vi "dsdll_basic_demo.vi"() -> ()   [LabVIEW 2013, in "dsdll.lvlib"]
doc: "Simple DSDLL demo. Allows to record waveform from selected source and than play it as loop."
uses:
  dsdll.lvlib
  dsdll_instance.ctl
  dsdll_device_record.ctl
  dsdll_format.ctl
  dsdll_sample_format.ctl
  output/dsdll_output_write_auto_float32.vi
  capture/dsdll_capture_wave_auto_float32.vi
panel:
  in  "gui refresh":i32=50 caption="GUI refresh [ms]"
  out "dsdll.dll version string":string
  out "play stat":i32(slide) scale=0.0..100.0
  out "invalid DSDLL instance handle?":bool
  out "output device ok?":bool
  out "output buffer ok?":bool
  out "input capture ok?":bool
  out "rec stat":i32(slide) scale=0.0..100.0
  out "stat str":string caption="Capture progress"
  out "is capturing?":bool
  in  "btn rec abort":bool
  out "record":sgl[][](graph)
  out "rec len out":u32 caption="Recorded samples"
  out "Time stamp [s]":dbl
  in  "btn rec":bool
  in  "btn stop":bool
  out "sound data":sgl[][](array[numeric])
  in  "format":T1={"sample rate [Hz]"=48000, "out channels"=1, "inp channels"=1, "format"=enum."IEEE float 32"} caption="Wave format"
  in  "btn close":bool
  in  "btn open":bool
  in  "btn exit":bool
  in  "rec len":u32=96000 caption="Samples count"
  in  "devs capt":u16(ring) caption="Capture devices" items=["Primarni ovladac pro digitalizaci zvuku", "Mikrofon (Zvukove zarizeni High Definition Audio)"]
  in  "devs out":u16(ring) caption="Output devices" items=["Primarni ovladac zvuku", "Reproduktory (Zvukove zarizeni High Definition Audio)"]
  in  "btn play":bool
  in  "btn enum":bool
  out "error out":errorcluster caption="Error out"
  out "dsdll":T3
  # "DirectSound DLL demo"
  # "1) select in/out devices\n2) select sample format\n3) open DSDLL instace\n4) record waveform\n5) play captured wave"
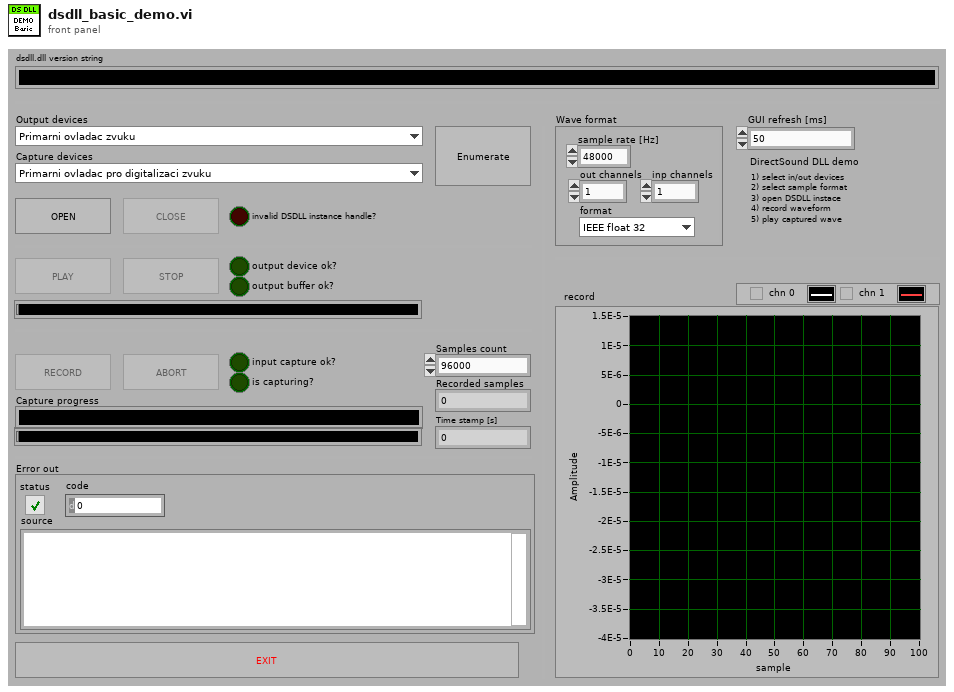
[diagram p1: front panel]
types:
  T1 = typedef "dsdll.lvlib/dsdll_format.ctl" = cluster{"sample rate [Hz]":u32, "out channels":u16, "inp channels":u16, "format":T2}
  T2 = typedef "dsdll.lvlib/dsdll_sample_format.ctl" = enum16{"IEEE float 32", "PCM 16 bit"}
  T3 = typedef "dsdll.lvlib/dsdll_instance.ctl" = cluster{"dsdll path":path, "dsdll handle":u8[], "output devices":T4[], "capture devices":T4[]}
  T4 = typedef "dsdll.lvlib/dsdll_device_record.ctl" = cluster{"guid":u8[], "name":string}
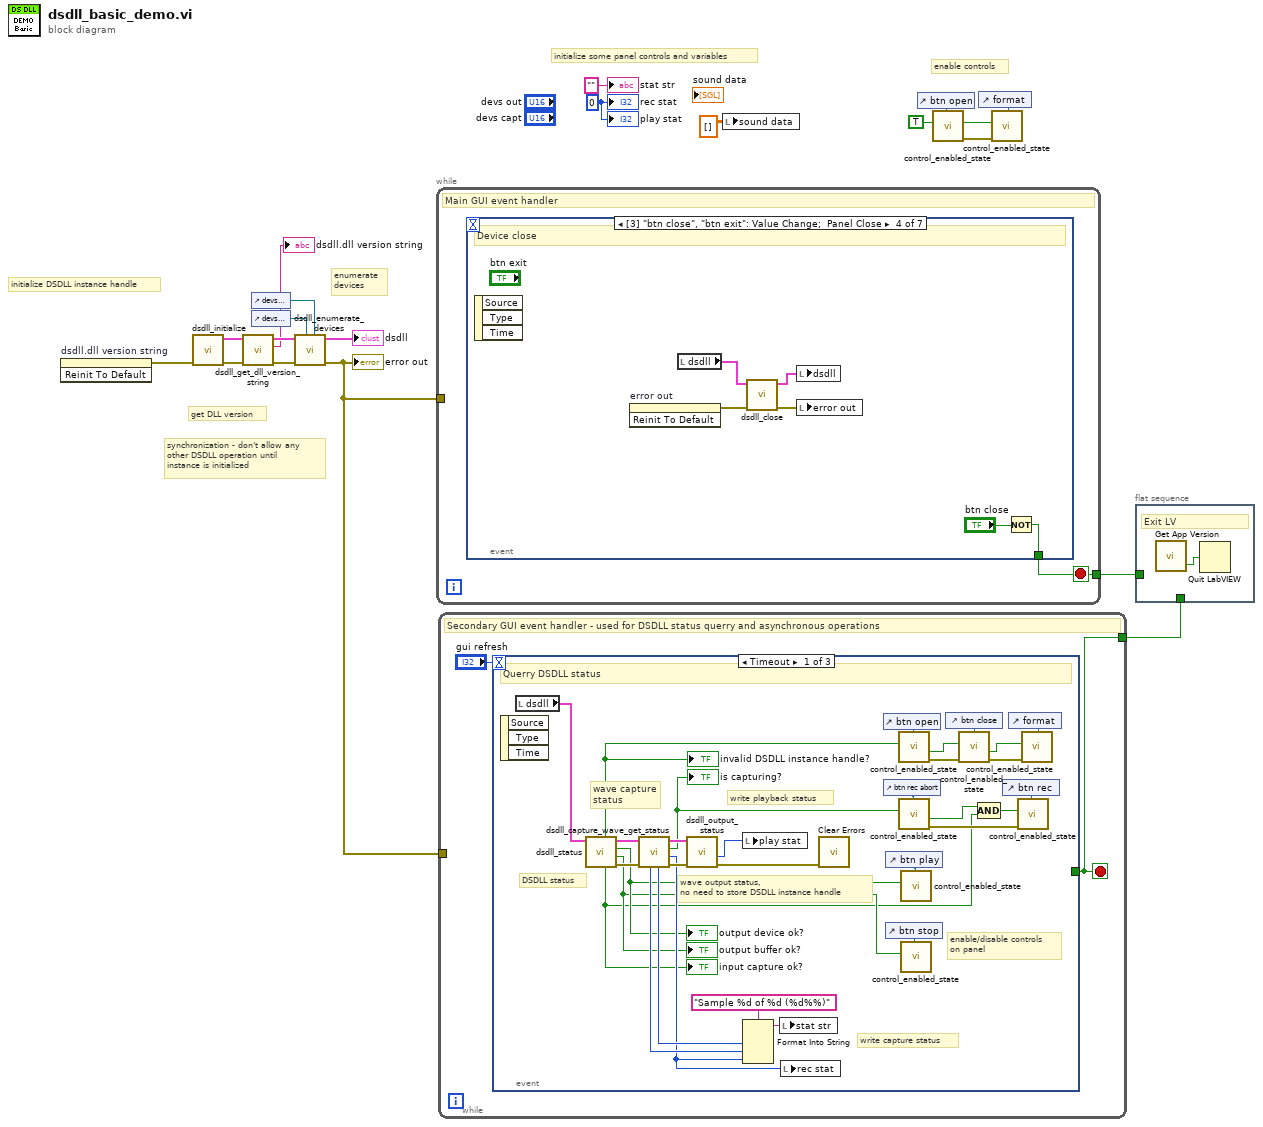
[diagram p0: block diagram]
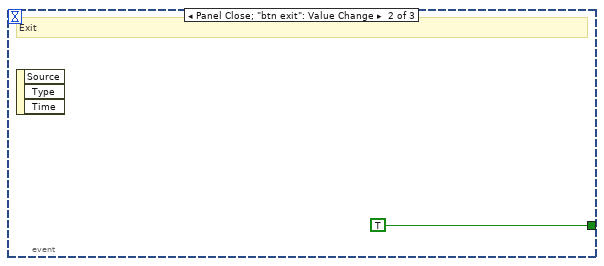
[diagram p2: hidden frame]
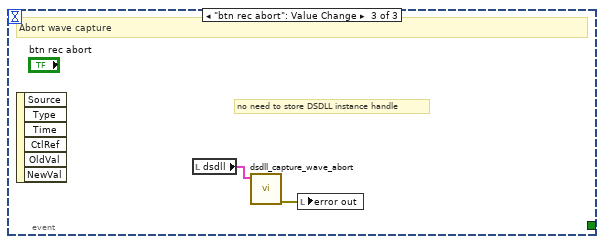
[diagram p3: hidden frame]
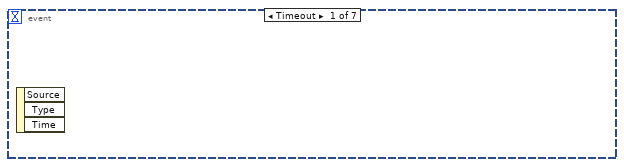
[diagram p4: hidden frame]
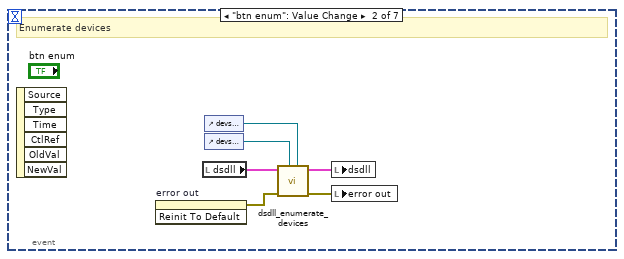
[diagram p5: hidden frame]
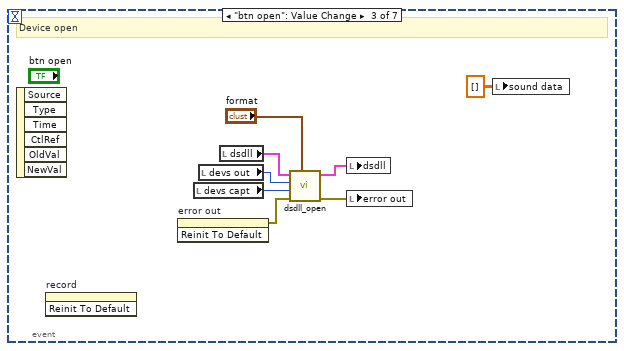
[diagram p6: hidden frame]
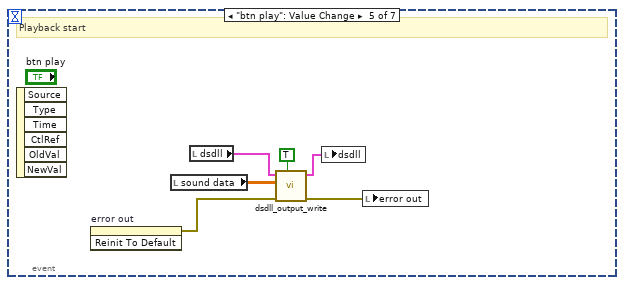
[diagram p7: hidden frame]
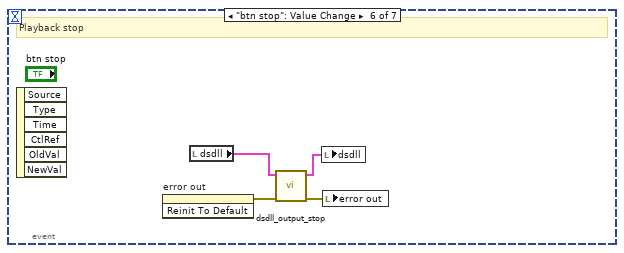
[diagram p8: hidden frame]
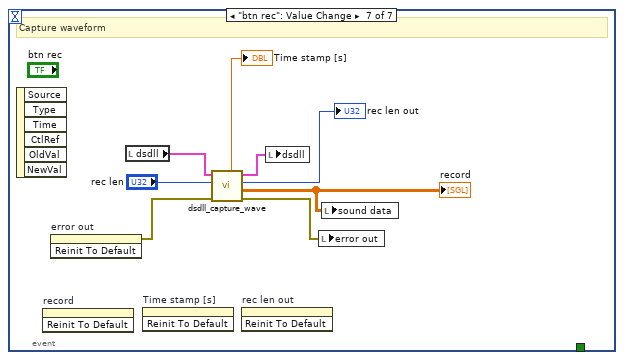
[diagram p9: hidden frame]
diagram:
  w14 = 0 ("rec stat")
  # "get DLL version"
  # "enumerate\ndevices"
  # "synchronization - don't allow any\nother DSDLL operation until\ninstance is initialized"
  # "initialize DSDLL instance handle"
  # "enable controls"
  # "initialize some panel controls and variables"
  n1 = invoke on="dsdll.dll version string" class="Str" method="Reinit To Default"() -> (error out=w2:errorcluster)  [unwired: 3 in, 2 out]
  n2 = call "dsdll_initialize.vi"("error in"=w2) -> ("error out"=w7:errorcluster, "dsdll instance out"=w5:T3)  [unwired: 9 in]
  n3 = call "dsdll_get_dll_version_string.vi"("error in"=w7, "dsdll instance in"=w5) -> ("error out"=w6:errorcluster, "version string"=→"dsdll.dll version string":string, "dsdll instance out"=w4:T3)  [unwired: 7 in]
  n4 = control-ref of="devs capt"() -> (w18:refnum<vi>)
  n5 = control-ref of="devs out"() -> (w19:refnum<vi>)
  n6 = call "dsdll_enumerate_devices.vi"("capture devices ring ref"=w18, "output devices ring ref"=w19, "error in"=w6, "dsdll instance in"=w4) -> ("error out"=w8:errorcluster, "dsdll instance out"=→"dsdll":T3)  [unwired: 4 in, 2 out]
  "error out" <- w8
  n7 = while {
    tunnel: [w21] -> w16
    tunnel: w8 -> [_]
    stop <- w21 stop-if-true
    # "Main GUI event handler"
    n8 = event shown="[3] \"btn close\", \"btn exit\": Value Change;  Panel Close" {
      selector: _ -> [_ _ _ _ _ _ _]
      dyn-events: _ -> [_ _ _ _ _ _ _]
      timeout: _ -> [_ _ _ _ _ _ _]
      tunnel: [_ _ _ w36 _ _ _] -> w21
      event Timeout {
        n9 = event-data() -> ()  [unwired: 1 in, 3 out]
      }
      event "btn enum": Value Change {
        # "Enumerate devices"
        n10 = event-data() -> ()  [unwired: 1 in, 6 out]
        n11 = invoke on="error out" class="Clust (strict)" method="Reinit To Default"() -> (error out=w22:errorcluster)  [unwired: 3 in, 2 out]
        n12 = local read "dsdll"() -> (w27:T3)
        n13 = control-ref of="devs capt"() -> (w24:refnum<vi>)
        n14 = control-ref of="devs out"() -> (w25:refnum<vi>)
        n15 = call "dsdll_enumerate_devices.vi"("capture devices ring ref"=w24, "output devices ring ref"=w25, "error in"=w22, "dsdll instance in"=w27) -> ("error out"=w26:errorcluster, "dsdll instance out"=w23:T3)  [unwired: 4 in, 2 out]
        n16 = local write "dsdll"(w23) -> ()
        n17 = local write "error out"(w26) -> ()
      }
      event "btn open": Value Change {
        # "Device open"
        n18 = event-data() -> ()  [unwired: 1 in, 6 out]
        n19 = invoke on="record" class="WFGraph (strict)" method="Reinit To Default"() -> ()  [unwired: 3 in, 3 out]
        n20 = invoke on="error out" class="Clust (strict)" method="Reinit To Default"() -> (error out=w31:errorcluster)  [unwired: 3 in, 2 out]
        n21 = local read "devs capt"() -> (w33:u16)
        n22 = local read "devs out"() -> (w32:u16)
        n23 = local read "dsdll"() -> (w35:T3)
        n24 = call "dsdll_open.vi"("format"="format", "error in"=w31, "capture device id"=w33, "output device id"=w32, "dsdll instance in"=w35) -> ("error out"=w30:errorcluster, "dsdll instance out"=w29:T3)  [unwired: 5 in]
        n25 = local write "dsdll"(w29) -> ()
        n26 = local write "error out"(w30) -> ()
        n27 = local write "sound data"(sgl[][] [] ("sound data")) -> ()
      }
      event "btn close", "btn exit": Value Change; Panel Close {
        # "Device close"
        n28 = event-data() -> ()  [unwired: 1 in, 3 out]
        n29 = invoke on="error out" class="Clust (strict)" method="Reinit To Default"() -> (error out=w38:errorcluster)  [unwired: 3 in, 2 out]
        n30 = local read "dsdll"() -> (w39:T3)
        n31 = call "dsdll_close.vi"("error in"=w38, "dsdll instance in"=w39) -> ("error out"=w41:errorcluster, "dsdll instance out"=w40:T3)  [unwired: 8 in]
        n32 = local write "dsdll"(w40) -> ()
        n33 = local write "error out"(w41) -> ()
        n34 = Not(x="btn close") -> (.not. x?=w36:bool)
      }
      event "btn play": Value Change {
        # "Playback start"
        n35 = event-data() -> ()  [unwired: 1 in, 6 out]
        n36 = invoke on="error out" class="Clust (strict)" method="Reinit To Default"() -> (error out=w46:errorcluster)  [unwired: 3 in, 2 out]
        n37 = local read "sound data"() -> (w42:sgl[][])
        n38 = local read "dsdll"() -> (w45:T3)
        n39 = call-poly "dsdll_output_write.vi"("play (true)"=TRUE ("play"), "error in"=w46, "float32 samples"=w42, "dsdll instance in"=w45) -> ("error out"=w43:errorcluster, "dsdll instance out"=w44:T3)  [unwired: 6 in]
        n40 = local write "dsdll"(w44) -> ()
        n41 = local write "error out"(w43) -> ()
      }
      event "btn stop": Value Change {
        # "Playback stop"
        n42 = event-data() -> ()  [unwired: 1 in, 6 out]
        n43 = invoke on="error out" class="Clust (strict)" method="Reinit To Default"() -> (error out=w51:errorcluster)  [unwired: 3 in, 2 out]
        n44 = local read "dsdll"() -> (w50:T3)
        n45 = call "dsdll_output_stop.vi"("error in"=w51, "dsdll instance in"=w50) -> ("error out"=w48:errorcluster, "dsdll instance out"=w49:T3)  [unwired: 8 in]
        n46 = local write "dsdll"(w49) -> ()
        n47 = local write "error out"(w48) -> ()
      }
      event "btn rec": Value Change {
        # "Capture waveform"
        n48 = event-data() -> ()  [unwired: 1 in, 6 out]
        n49 = invoke on="record" class="WFGraph (strict)" method="Reinit To Default"() -> ()  [unwired: 3 in, 3 out]
        n50 = invoke on="error out" class="Clust (strict)" method="Reinit To Default"() -> (error out=w59:errorcluster)  [unwired: 3 in, 2 out]
        n51 = local read "dsdll"() -> (w58:T3)
        n52 = invoke on="Time stamp [s]" class="DigNum (strict)" method="Reinit To Default"() -> ()  [unwired: 3 in, 3 out]
        n53 = call-poly "dsdll_capture_wave.vi"("error in"=w59, "samples count in"="rec len", "dsdll instance in"=w58) -> ("error out"=w56:errorcluster, "float32 waves"=w52:sgl[][], "samples count out"=→"rec len out":u32, "dsdll instance out"=w57:T3, "time stamp [s]"=→"Time stamp [s]":dbl)  [unwired: 3 in, 1 out]
        "record" <- w52
        n54 = invoke on="rec len out" class="DigNum (strict)" method="Reinit To Default"() -> ()  [unwired: 3 in, 3 out]
        n55 = local write "dsdll"(w57) -> ()
        n56 = local write "error out"(w56) -> ()
        n57 = local write "sound data"(w52) -> ()
      }
    }
  }
  n58 = while {
    tunnel: w8 -> [_]
    tunnel: [w60] -> w1
    stop <- w60 stop-if-true
    # "Secondary GUI event handler - used for DSDLL status querry and asynchronous operations"
    n59 = event shown="[0] Timeout" {
      selector: _ -> [_ _ _]
      dyn-events: _ -> [_ _ _]
      timeout: "gui refresh" -> [_ _ _]
      tunnel: [_ TRUE _] -> w60
      event Timeout {
        # "wave capture\nstatus"
        # "DSDLL status"
        # "wave output status,\nno need to store DSDLL instance handle"
        # "write playback status"
        # "write capture status"
        # "enable/disable controls\non panel"
        # "Querry DSDLL status"
        n60 = event-data() -> ()  [unwired: 1 in, 3 out]
        n61 = local read "dsdll"() -> (w87:T3)
        n62 = call "dsdll_status.vi"("dsdll instance in"=w87) -> ("error out"=w88:errorcluster, "output buffer ok"=w68:bool, "output device ok"=w70:bool, "dsdll instance out"=w86:T3, "input capture ok"=w65:bool, "invalid instance handle"=w76:bool)  [unwired: 5 in]
        "input capture ok?" <- w65
        "output buffer ok?" <- w68
        "output device ok?" <- w70
        "invalid DSDLL instance handle?" <- w76
        n63 = call "dsdll_capture_wave_get_status.vi"("error in"=w88, "dsdll instance in"=w86) -> ("error out"=w89:errorcluster, "progress [%]"=w82:i32, "is capturing?"=w74:bool, "dsdll instance out"=w85:T3, "actual sample position"=w91:u32, "total samples count"=w90:u32)  [unwired: 4 in]
        "is capturing?" <- w74
        n64 = call "dsdll_output_status.vi"("error in"=w89, "dsdll instance in"=w85) -> ("error out"=w84:errorcluster, "cursor position [%]"=w81:i32)  [unwired: 3 in, 5 out]
        n65 = local write "play stat"(w81) -> ()
        n66 = Format Into String(format string="Sample %d of %d (%d%%)", w91, w90, w82) -> (resulting string=w83:string)  [unwired: 2 in, 1 out]
        n67 = local write "stat str"(w83) -> ()
        n68 = local write "rec stat"(w82) -> ()
        n69 = call <vilib>:"Clear Errors.vi"("error in (no error)"=w84) -> ()  [unwired: 6 in, 1 out]
        n70 = control-ref of="btn open"() -> (w80:refnum<vi>)
        n71 = control-ref of="btn rec abort"() -> (w75:refnum<vi>)
        n72 = control-ref of="btn play"() -> (w71:refnum<vi>)
        n73 = control-ref of="btn stop"() -> (w69:refnum<vi>)
        n74 = call "control_enabled_state.vi"("enabled"=w76, "control in"=w80) -> ("error out"=w79:errorcluster, "disabled"=w77:bool)  [unwired: 6 in, 2 out]
        n75 = call "control_enabled_state.vi"("enabled"=w74, "control in"=w75) -> ("error out"=w72:errorcluster, "disabled"=w66:bool)  [unwired: 6 in, 2 out]
        n76 = call "control_enabled_state.vi"("enabled"=w70, "control in"=w71) -> ()  [unwired: 6 in, 4 out]
        n77 = call "control_enabled_state.vi"("enabled"=w68, "control in"=w69) -> ()  [unwired: 6 in, 4 out]
        n78 = control-ref of="btn close"() -> (w78:refnum<vi>)
        n79 = call "control_enabled_state.vi"("error in (no error)"=w79, "enabled"=w77, "control in"=w78) -> ("error out"=w64:errorcluster, "disabled"=w62:bool)  [unwired: 5 in, 2 out]
        n80 = Compound Arithmetic op=AND(w66, w65) -> (w67:bool)
        n81 = control-ref of="btn rec"() -> (w73:refnum<vi>)
        n82 = control-ref of="format"() -> (w63:refnum<vi>)
        n83 = call "control_enabled_state.vi"("error in (no error)"=w72, "enabled"=w67, "control in"=w73) -> ()  [unwired: 5 in, 4 out]
        n84 = call "control_enabled_state.vi"("error in (no error)"=w64, "enabled"=w62, "control in"=w63) -> ()  [unwired: 5 in, 4 out]
      }
      event Panel Close; "btn exit": Value Change {
        # "Exit"
        n85 = event-data() -> ()  [unwired: 1 in, 3 out]
      }
      event "btn rec abort": Value Change {
        # "no need to store DSDLL instance handle"
        # "Abort wave capture"
        n86 = event-data() -> ()  [unwired: 1 in, 6 out]
        n87 = local read "dsdll"() -> (w94:T3)
        n88 = call "dsdll_capture_wave_abort.vi"("dsdll instance in"=w94) -> ("error out"=w95:errorcluster)  [unwired: 8 in, 2 out]
        n89 = local write "error out"(w95) -> ()
      }
    }
  }
  n90 = local write "sound data"(sgl[][] [] ("sound data")) -> ()
  n91 = control-ref of="btn open"() -> (w12:refnum<vi>)
  n92 = call "control_enabled_state.vi"("enabled"=TRUE, "control in"=w12) -> ("error out"=w10:errorcluster, "enabled"=w9:bool)  [unwired: 6 in, 2 out]
  n93 = control-ref of="format"() -> (w11:refnum<vi>)
  n94 = call "control_enabled_state.vi"("error in (no error)"=w10, "enabled"=w9, "control in"=w11) -> ()  [unwired: 5 in, 4 out]
  n95 = flat-sequence {
    tunnel: w16 -> [_]
    tunnel: w1 -> [_]
    frame #0 {
      # "Exit LV"
      n96 = call "Get App Version.vi"() -> ("runtime"=w96:bool)  [unwired: 1 out]
      n97 = Quit LabVIEW(quit? (T)=w96) -> ()
    }
  }
  "rec stat" <- w14
  "stat str" <- "" ("stat str")
  "play stat" <- w14
